vi "prepare connection.vi"(7 "client string":string, 8 "error in":errorcluster, 9 "connection string":string, 10 "to queue manager":refnum<queue>, 11 "connection in":refnum<class "connection maintainer.lvclass">) -> (0 "error out":errorcluster, 3 "connection out":refnum<class "connection maintainer.lvclass">)   [LabVIEW 2015, in "connection maintainer.lvclass"]
uses:
  connection maintainer.lvclass
  message/communicator message.lvclass
  connection maintainer.lvclass/connection maintainer.ctl
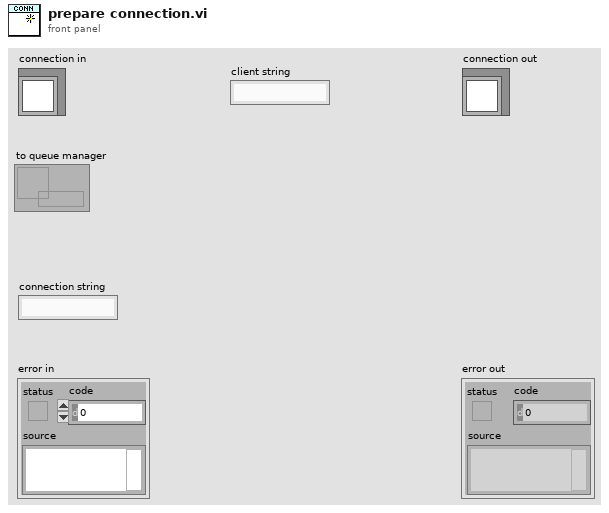
[diagram p1: front panel]
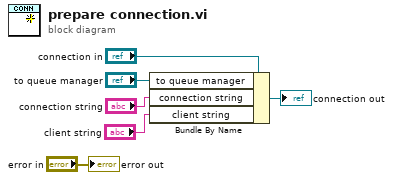
[diagram p0: block diagram]
diagram:
  n1 = Bundle By Name(cluster="connection in", "to queue manager"="to queue manager", "connection string"="connection string", "client string"="client string") -> (→"connection out":refnum<class "connection maintainer.lvclass">)
  "error out" <- "error in"
